vi "wrapper.vi"(1 "Parameter":variant[](array[variant])) -> (0 "Result":variant[](array[variant]))   [LabVIEW 2012]
panel:
  out "data":u32
  out "SetupID":u32
  out "waveformType":string
  out "samplingTime":dbl
  out "samplingRate":u32
  out "offset":dbl
  out "amplitude":dbl
  out "frequency":dbl
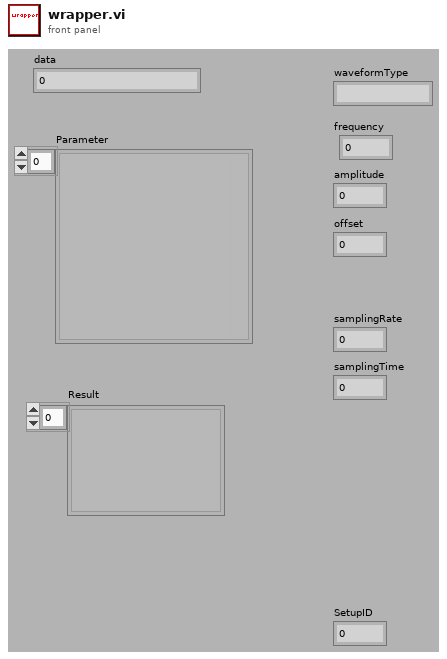
[diagram p1: front panel]
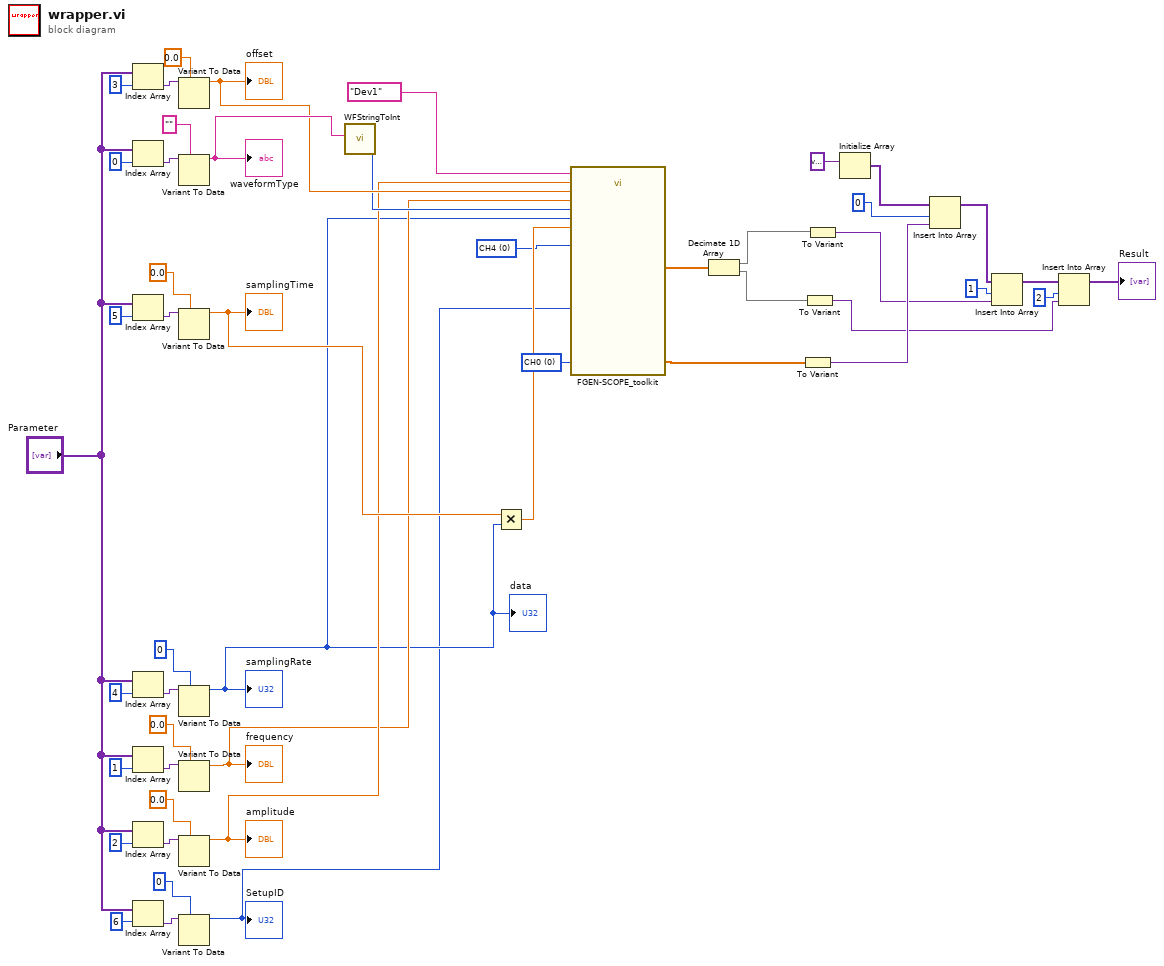
[diagram p0: block diagram]
diagram:
  w1 = u16 0 items=["CH4", "CH5", "CH6", "CH7"] ("ChB_Source")
  w2 = u16 0 items=["CH0", "CH1", "CH2", "CH3"] ("ChA_Source")
  n1 = Index Array(array="Parameter", index=3) -> (element=w42:variant)
  n2 = Index Array(array="Parameter", index=0) -> (element=w39:variant)
  n3 = Index Array(array="Parameter", index=5) -> (element=w34:variant)
  n4 = Index Array(array="Parameter", index=4) -> (element=w37:variant)
  n5 = Index Array(array="Parameter", index=1) -> (element=w48:variant)
  n6 = Index Array(array="Parameter", index=2) -> (element=w45:variant)
  n7 = Index Array(array="Parameter", index=6) -> (element=w30:variant)
  n8 = Variant To Data(type=0.0 ("double precision float"), Variant=w42) -> (data=w9:dbl)  [unwired: 1 in, 1 out]
  "offset" <- w9
  n9 = Variant To Data(type="", Variant=w39) -> (data=w31:string)  [unwired: 1 in, 1 out]
  "waveformType" <- w31
  n10 = Variant To Data(type=0.0 ("double precision float"), Variant=w34) -> (data=w11:dbl)  [unwired: 1 in, 1 out]
  "samplingTime" <- w11
  n11 = Variant To Data(type=u32 0 ("double precision float"), Variant=w37) -> (data=w5:u32)  [unwired: 1 in, 1 out]
  "samplingRate" <- w5
  "data" <- w5
  n12 = Variant To Data(type=0.0 ("double precision float"), Variant=w48) -> (data=w6:dbl)  [unwired: 1 in, 1 out]
  "frequency" <- w6
  n13 = Variant To Data(type=0.0 ("double precision float"), Variant=w45) -> (data=w7:dbl)  [unwired: 1 in, 1 out]
  "amplitude" <- w7
  n14 = Variant To Data(type=u32 0 ("double precision float"), Variant=w30) -> (data=w4:u32)  [unwired: 1 in, 1 out]
  "SetupID" <- w4
  n15 = call "WFStringToInt.vi"("WaveFormType"=w31) -> ("WaveFormTypeInt"=w8:u16)  [unwired: 10 in]
  n16 = Multiply(x=w11, y=w5) -> (x*y=w19:dbl)
  n17 = call "FGEN-SCOPE_toolkit.vi"("Device Name"=tag "Dev1", "Amplitude"=w7, "DC Offset"=w9, "Frequency"=w6, "Waveform Type"=w8, "Sample Rate (Hz)"=w5, "Record Length"=w19, "ChA_Source"=w2, "ChB_Source"=w1, "SetupID"=w4) -> ("interleaved array"=w17:dbl[], "time vector"=w18:dbl[])  [unwired: 15 in, 1 out]
  n18 = Decimate 1D Array(w17) -> (w16:dbl[], w15:dbl[])
  n19 = To Variant(anything=w18) -> (Variant=w14:variant)
  n20 = To Variant(anything=w15) -> (Variant=w12:variant)
  n21 = To Variant(anything=w16) -> (Variant=w13:variant)
  n22 = Initialize Array(variant ("variant")) -> (w25:variant[])  [unwired: 1 in]
  n23 = Insert Into Array(array=w25, index=0, new element=w14) -> (w24:variant[])
  n24 = Insert Into Array(array=w24, index=1, new element=w13) -> (w22:variant[])
  n25 = Insert Into Array(array=w22, index=2, new element=w12) -> (→"Result":variant[])
